vi "3DS Scene.vi"(8 "error in (no error)":errorcluster, 9 "Draw Style:Mode":T1(ring)=enum."Wireframe", 11 "SceneMesh in":refnum<vi>) -> (0 "error out":errorcluster, 3 "SceneObject out":refnum<vi>)   [LabVIEW 2026, in "3D utilities.lvlib"]
uses:
  3D utilities.lvlib
  <vilib>/picture/3D Picture Control/Object/Create Object (name).vi
  <vilib>/picture/3D Picture Control/NI_3D Picture Control.lvlib
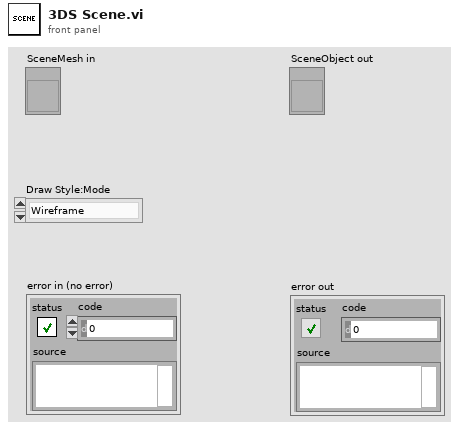
[diagram p1: front panel]
types:
  T1 = enum16{"Inherit Value", "Points", "Wireframe", "Polygons"}
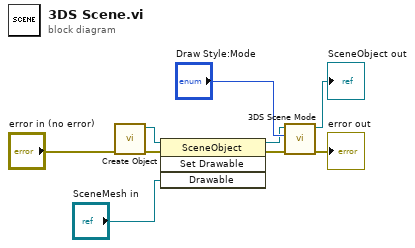
[diagram p0: block diagram]
diagram:
  n1 = call-poly <vilib>:"Create Object.vi"("error in (no error)"="error in (no error)") -> ("error out"=w3:errorcluster, "Scene:New Object"=w6:refnum<vi>)  [unwired: 9 in]
  n2 = invoke class="SceneObject" method="Set Drawable"(reference=w6, error in=w3, "Drawable"="SceneMesh in") -> (reference out=w5:refnum<vi>, error out=w2:errorcluster)  [unwired: 1 in, 2 out]
  n3 = call "3DS Scene Mode.vi"("error in (no error)"=w2, "Draw Style:Mode"="Draw Style:Mode", "SceneObject in"=w5) -> ("error out"=→"error out":errorcluster, "SceneObject out"=→"SceneObject out":refnum<vi>)  [unwired: 7 in]
